vi "ACC_MANAGEMENT.vi"() -> ()   [LabVIEW 2018]
uses:
  <vilib>/addons/database/Connection.llb/DB Tools Open Connec (Path).vi
  <vilib>/addons/database/Connection.llb/Conn Execute.vi
  <vilib>/addons/database/Recordset.llb/Rec Fetch Recordset Data (R).vi
  <vilib>/addons/database/Recordset.llb/Rec Destroy - Connection.vi
  <vilib>/addons/database/_DB Variant To Data/Database Variant To Data.xnode
  <vilib>/addons/database/NI_Database_API.lvlib
panel:
  in  "MAIN_TAB":T1(tab)
  in  "ACC_PASSPORT_VALID":string caption="NEW PASSWORD"
  in  "ACC_SAVE":bool
  in  "ACC_IMG_UP":bool
  in  "ACC_STAMP":string caption="SUPPORTING"
  in  "ACC_TITLE":string caption="NEW PASSWORD"
  in  "ACC_UNIT":string caption="NEW PASSWORD"
  in  "ACC_EMAIL":string caption="NEW PASSWORD"
  in  "ACC_NAME":string caption="NEW PASSWORD"
  in  "ACC_UID":string caption="CONFIRM NEW PASSWORD"
  out "ACC_ACCESS":string[][](table)
  in  "ACC_BUTTON1":bool
  in  "ACC_PSW2":string caption="CONFIRM PASSWORD"
  in  "ACC_PSW1":string caption="NEW PASSWORD"
  in  "ACC_OPTION":enum32{"Item 0", "Item 1", "Item 2"}(radio)
  out "ACC_IMG":picture
  in  "ACC_IMG_DN":bool
  in  "ACC_BUTTON2":bool
  in  "ACC_STAMP_STATUS":bool
  out "ACC_STATUS":bool caption="TRANSACTION SUCCESS"
  in  "ACC_TAG":u16(ring) items=["BARCODE", "RFID", "NFC"]
  out "ACC_TAG_ID":string caption="NEW PASSWORD"
  in  "ACC_PASSPORT_UP":bool
  in  "ACC_PASSPORT_DN":bool
  in  "ACC_PASSPORT":string caption="NEW PASSWORD"
  in  "ACC_PASSPORT_TIMESTAMP":timestamp format="%<%b %d, %Y>T"
  in  "ACC_PASSPORT_STATUS":bool
  in  "MNG_MODULE_ACC":u16(ring) items=["R", "R/W", "R/W/D"]
  in  "MNG_MODULE":i32(listbox)
  in  "MNG_KEYWORD":string
  in  "MNG_SELECT":u16(ring) items=["by UID", "by NAME", "by EMAIL"]
  out "MNG_STATUS":bool
  in  "MNG_SRC/DLT":bool
  in  "MNG_MODULE_UPD":bool
  out "MAIN_NOTE":string caption="ADDITIONAL NOTE :"
  in  "MAIN_CLOSE":bool
  in  "MAIN_LOGIN":string
  # "ACCOUNT MANAGEMENT"
  # "UID :"
  # "PSW :"
  # "BASIC INFORMATION"
  # "NAME   :"
  # "EMAIL  :"
  # "UNIT   :"
  # "TITLE  :"
  # "STAMP  :"
  # "SMART TAG"
  # ":"
  # "TRAVEL DOCUMENT"
  # "PASSPORT    :"
  # "VALID UNTIL :"
  # "ACCESSIBILITY :"
  # "KEYWORD :"
  # "ACCESSIBILITY :"
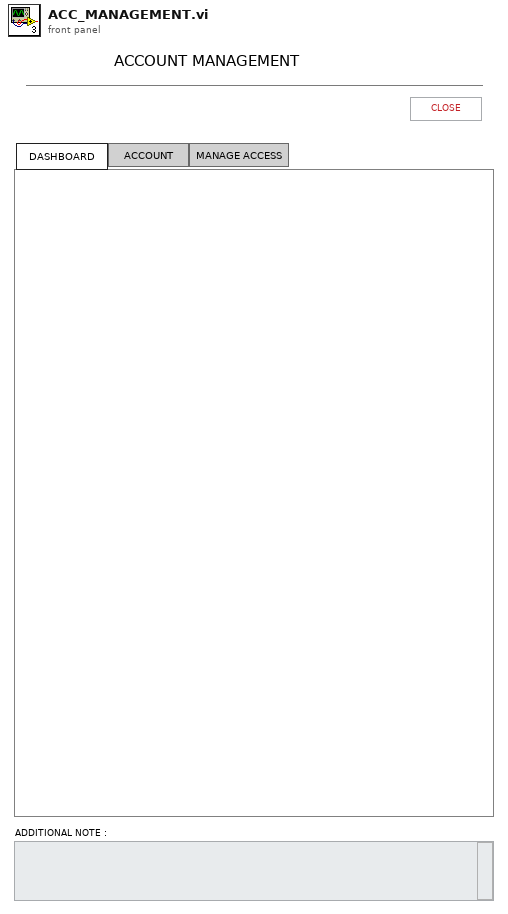
[diagram p1: front panel]
types:
  T1 = enum32{"DASHBOARD    ", "ACCOUNT      ", "MANAGE ACCESS"}
  T2 = enum16{"open", "replace", "create", "open or create", "replace or create", "replace or create with confirmation"}
  T3 = enum8{"Enabled", "Disabled", "Disabled and Grayed Out"}
  T4 = typedef "NI_Database_API.lvlib/Conn ObjectReference.ctl" = refnum<k1>
  T5 = typedef "NI_Database_API.lvlib/Rec ObjectReference.ctl" = refnum<k1>
  T6 = cluster{string[], string[], string[], string[], string[], path, path}
  T7 = typedef "LVBoundsTypeDef.ctl" = cluster{"Width":u32, "Height":u32}
  T8 = typedef "imagedata.ctl" = cluster{"image type":i32, "image depth":i32, "image":u8[], "mask":u8[], "colors":u32[], "Rectangle":cluster{"left":i16, "top":i16, "right":i16, "bottom":i16}}
  T9 = cluster{string[], string[], string[], string[], string[], "new picture":picture, dbl, bool}
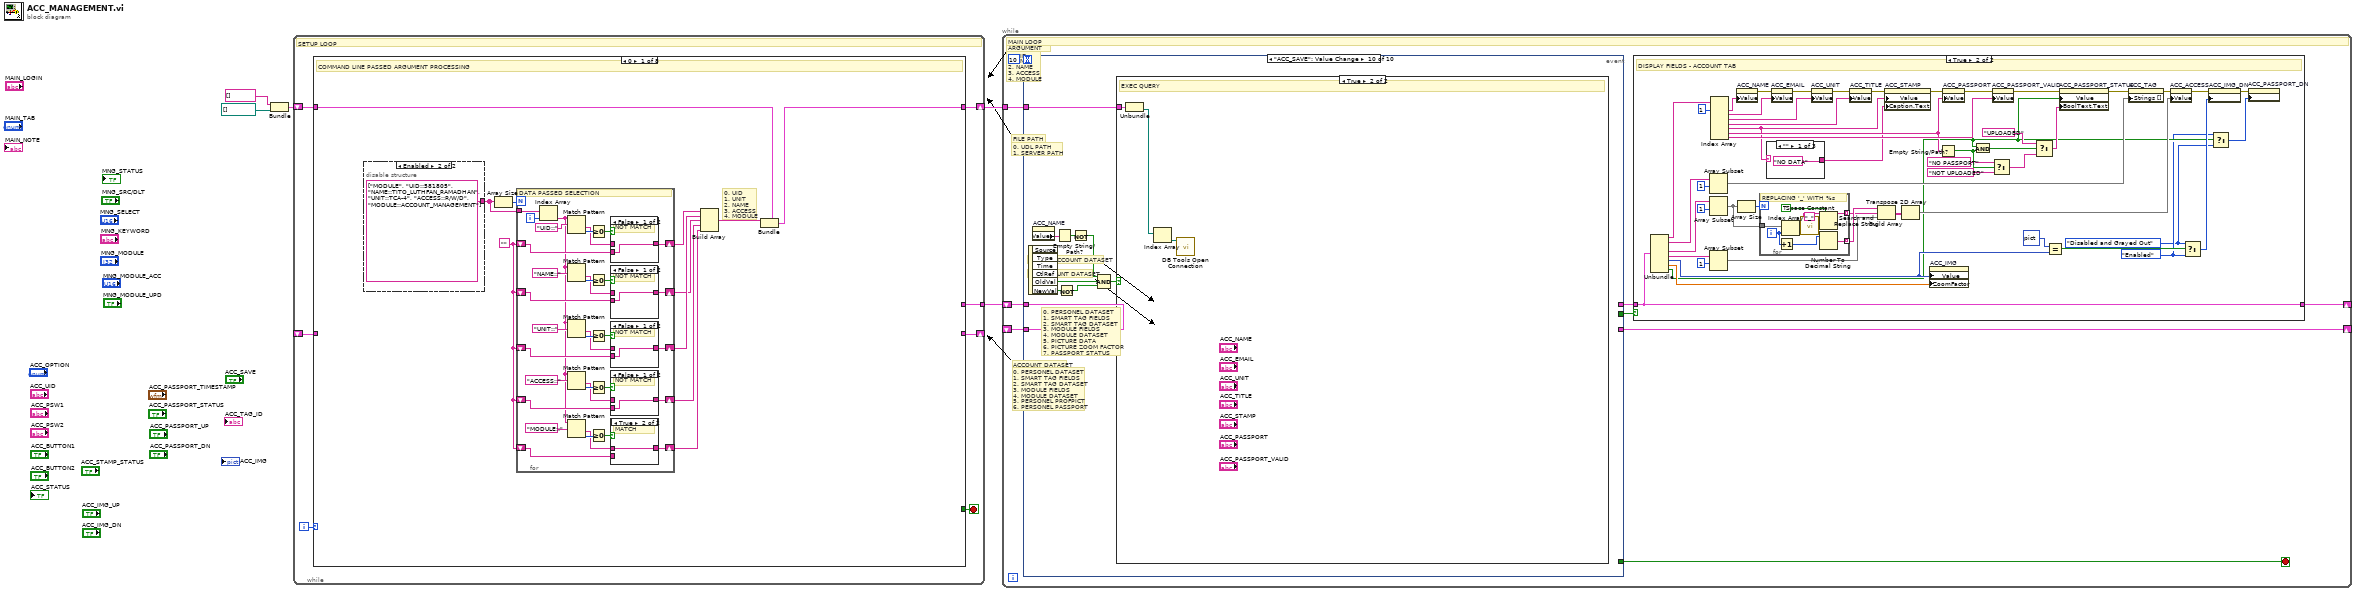
[diagram p0: block diagram]
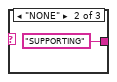
[diagram p3: hidden frame]
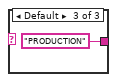
[diagram p4: hidden frame]
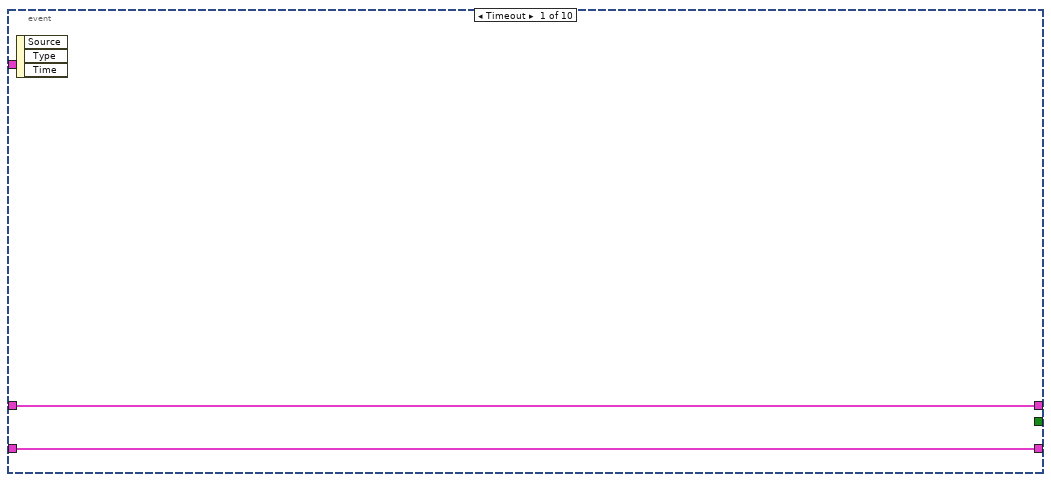
[diagram p5: hidden frame]
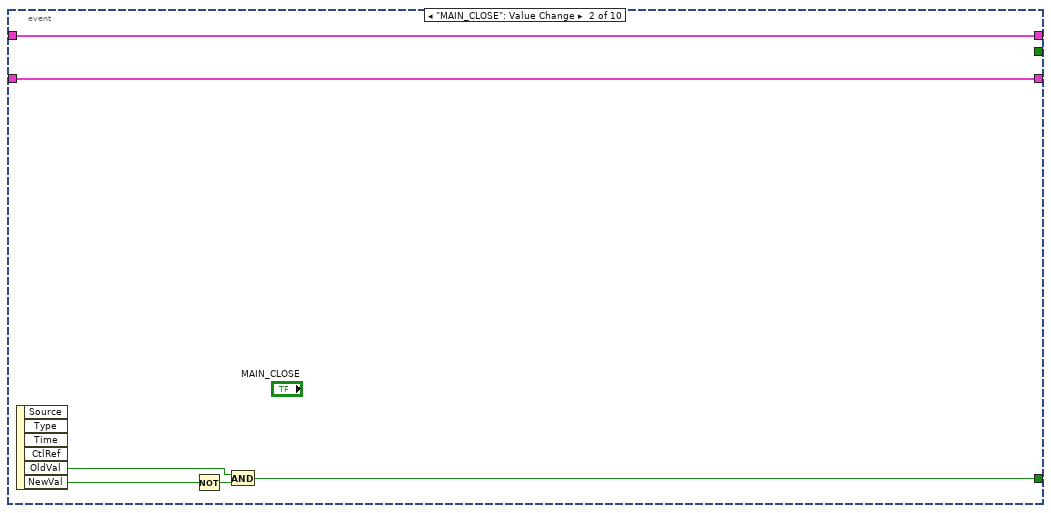
[diagram p6: hidden frame]
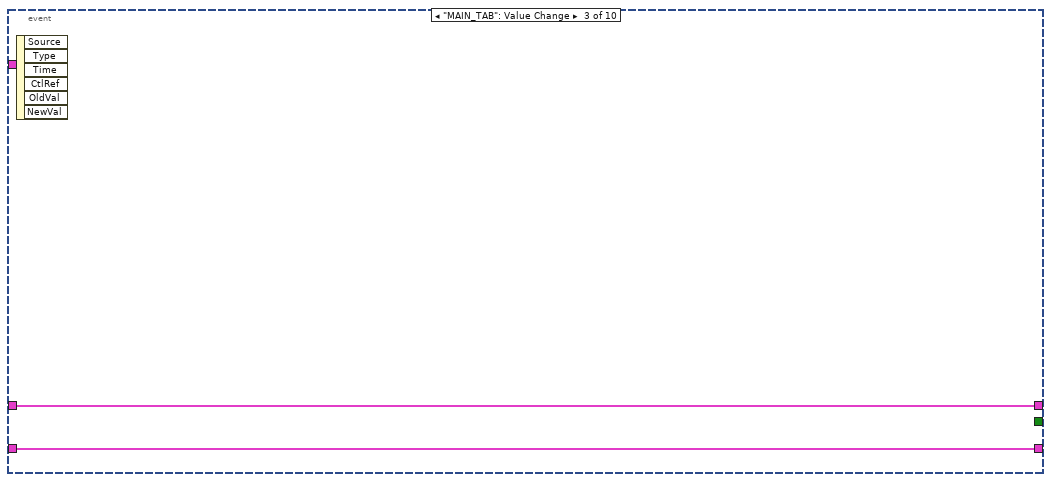
[diagram p7: hidden frame]
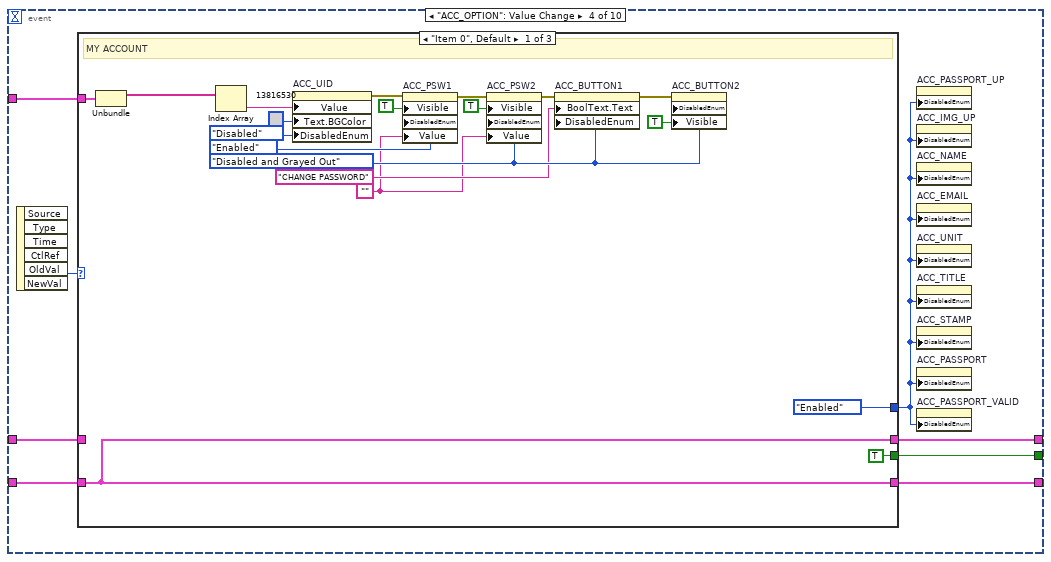
[diagram p8: hidden frame]
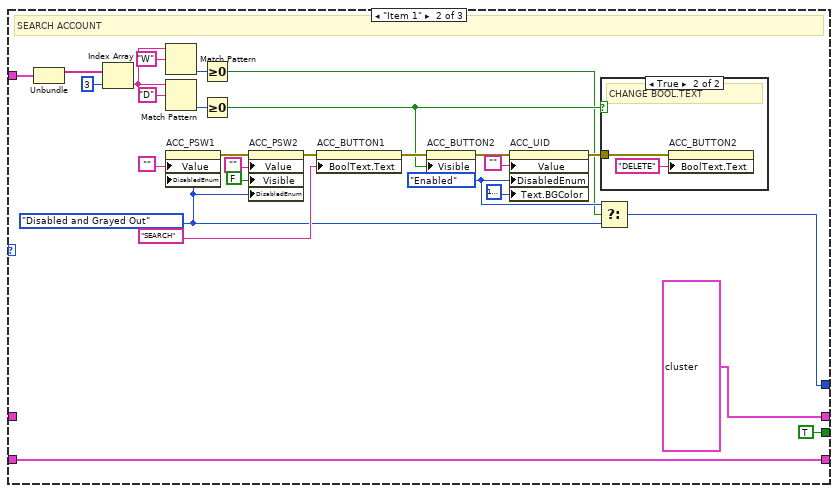
[diagram p9: hidden frame]
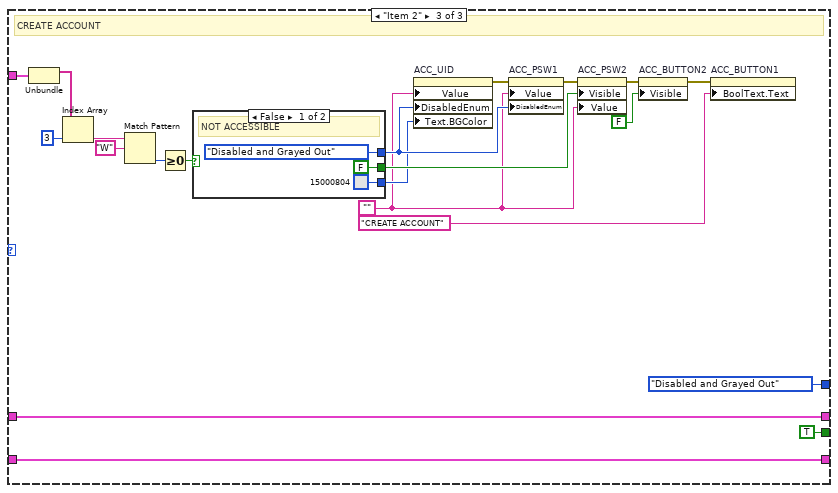
[diagram p11: hidden frame]
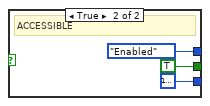
[diagram p12: hidden frame]
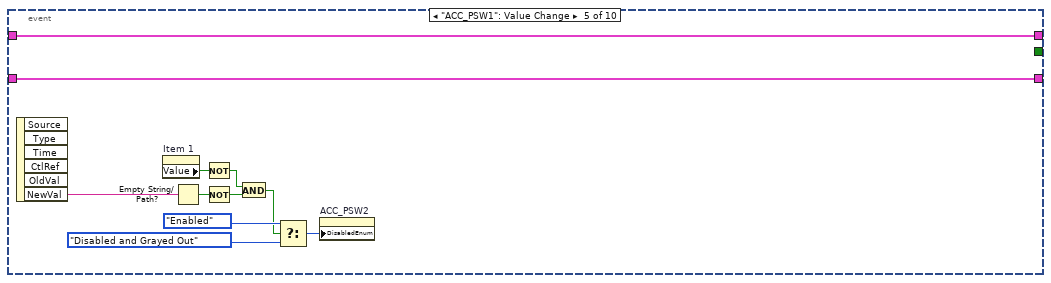
[diagram p13: hidden frame]
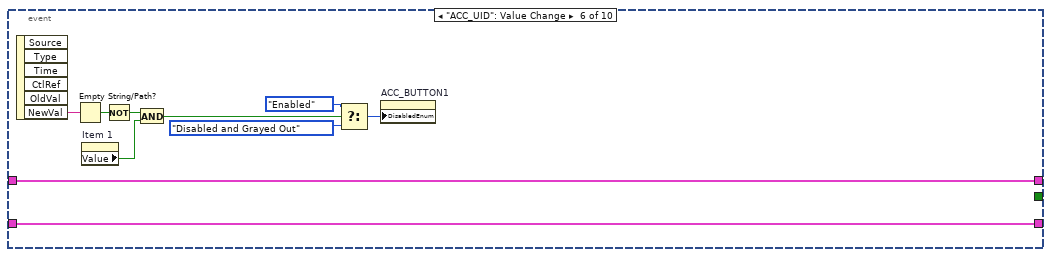
[diagram p14: hidden frame]
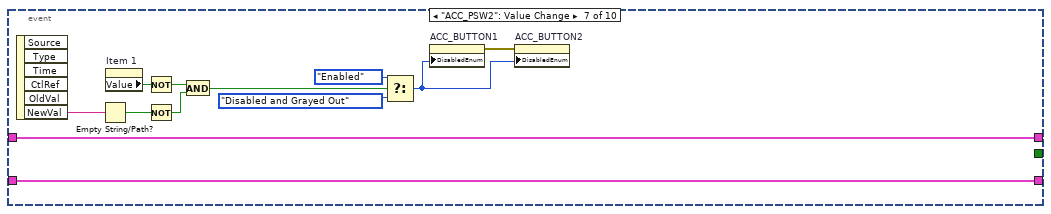
[diagram p15: hidden frame]
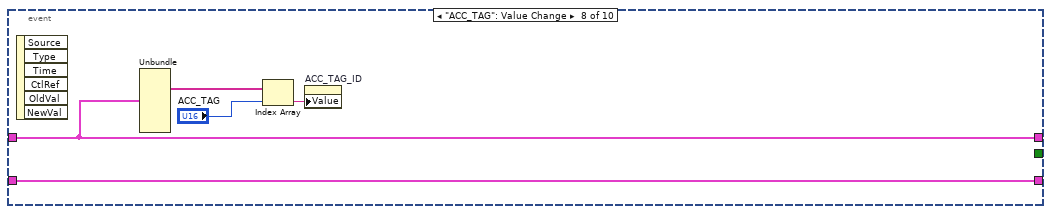
[diagram p16: hidden frame]
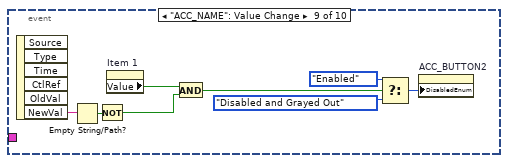
[diagram p17: hidden frame]
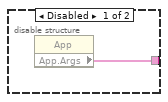
[diagram p19: hidden frame]
diagram:
  # "MY ACCOUNT DATASET"
  # "0. PERSONEL DATASET\n1. SMART TAG FIELDS\n2. SMART TAG DATASET\n3. MODULE FIELDS\n4. MODULE DATASET\n5. PICTURE DATA\n6. PICTURE ZOOM FACTOR\n7. PASSPORT STATUS"
  # "OTHER ACCOUNT DATASET"
  # "0. PERSONEL DATASET\n1. SMART TAG FIELDS\n2. SMART TAG DATASET\n3. MODULE FIELDS\n4. MODULE DATASET\n5. PERSONEL PROFPICT\n6. PERSONEL PASSPORT"
  # "0. UDL PATH\n1. SERVER PATH"
  # "0. UID\n1. UNIT\n2. NAME\n3. ACCESS\n4. MODULE"
  # "ACCOUNT DATASET"
  # "FILE PATH"
  # "COMMAND LINE\nARGUMENT"
  n1 = Bundle(string[] [], path[] []) -> (w3:cluster{string[], path[]})  [unwired: 1 in]
  n2 = while {
    shift-right: [w11] -> _
    shift-left: _ -> [w10]
    tunnel: [w8] -> w1
    shift-right: [w7] -> w2
    shift-left: w3 -> [w6]
    i -> [w12]
    stop <- w9 stop-if-true
    # "SETUP LOOP"
    n3 = case shown="0" w12 {
      tunnel: [_ _ _ w163 _ _ _ TRUE] -> w9
      tunnel: [_ _ _ w157 w405 w500 w523 w532] -> w11
      tunnel: w10 -> [_ _ _ w156 w405 w500 w523 w532]
      tunnel: [_ _ _ _ _ _ _ w531] -> w8
      tunnel: w6 -> [w15 w73 w98 w155 w404 w408 w522 w530]
      tunnel: [w13 w73 w96 w155 w404 w408 w522 w530] -> w7
      frame 0 {
        w21 = ""
        # "0. UID\n1. UNIT\n2. NAME\n3. ACCESS\n4. MODULE"
        # "COMMAND LINE PASSED ARGUMENT PROCESSING"
        n4 = disable-structure shown="Enabled" {
          disable-tunnel: [w24 string[] ["MODULE", "UID::581805", "NAME::TITO_LUTHFAN_RAMADHAN", "UNIT::TCA-4", "ACCESS::R/W/D", "MODULE::ACCOUNT_MANAGEMENT"] ("App.Args")] -> w22
          frame Disabled {
            n5 = property class="App"() -> ("App.Args"=w24:string[])  [unwired: 2 in, 2 out]
          }
          frame Enabled {
          }
        }
        n6 = Array Size(array=w22) -> (size(s)=w23:i32)
        n7 = for {
          N: w23 -> [_]
          tunnel: w22 -> [w58]
          shift-right: [w52] -> w19
          shift-left: w21 -> [w47]
          shift-right: [w46] -> w17
          shift-left: w21 -> [w45]
          shift-right: [w41] -> w18
          shift-left: w21 -> [w39]
          shift-right: [w34] -> w16
          shift-left: w21 -> [w33]
          shift-right: [w28] -> w20
          shift-left: w21 -> [w27]
          i -> [w57]
          # "DATA PASSED SELECTION"
          n8 = Index Array(array=w58, index=w57) -> (element=w26:string)
          n9 = Match Pattern(string=w26, regular expression="UID::") -> (after substring=w53:string, offset past match=w55:i32)  [unwired: 1 in, 2 out]
          n10 = Match Pattern(string=w26, regular expression="NAME::") -> (after substring=w48:string, offset past match=w51:i32)  [unwired: 1 in, 2 out]
          n11 = Match Pattern(string=w26, regular expression="UNIT::") -> (after substring=w40:string, offset past match=w44:i32)  [unwired: 1 in, 2 out]
          n12 = Match Pattern(string=w26, regular expression="ACCESS::") -> (after substring=w35:string, offset past match=w37:i32)  [unwired: 1 in, 2 out]
          n13 = Match Pattern(string=w26, regular expression="MODULE::") -> (after substring=w29:string, offset past match=w31:i32)  [unwired: 1 in, 2 out]
          n14 = Greater Or Equal To 0?(x=w55) -> (x >= 0?=w54:bool)
          n15 = Greater Or Equal To 0?(x=w51) -> (x >= 0?=w50:bool)
          n16 = Greater Or Equal To 0?(x=w44) -> (x >= 0?=w43:bool)
          n17 = Greater Or Equal To 0?(x=w37) -> (x >= 0?=w38:bool)
          n18 = Greater Or Equal To 0?(x=w31) -> (x >= 0?=w32:bool)
          n19 = case shown="False" w54 {
            tunnel: [w71 w72] -> w52
            tunnel: w53 -> [_ w72]
            tunnel: w47 -> [w71 _]
            frame False {
              # "NOT MATCH"
            }
            frame True {
              # "MATCH"
            }
          }
          n20 = case shown="False" w50 {
            tunnel: [w65 w66] -> w46
            tunnel: w48 -> [_ w70]
            tunnel: w45 -> [w65 _]
            frame False {
              # "NOT MATCH"
            }
            frame True {
              # "MATCH"
              n21 = call <vilib>:"Space Constant.vi"() -> ("String"=w68:string)
              n22 = Search and Replace String(replace all?=TRUE ("replace all? (F)"), input string=w70, search string="_", replace string=w68) -> (result string=w66:string)  [unwired: 4 in, 3 out]
            }
          }
          n23 = case shown="False" w43 {
            tunnel: [w63 w64] -> w41
            tunnel: w40 -> [_ w64]
            tunnel: w39 -> [w63 _]
            frame False {
              # "NOT MATCH"
            }
            frame True {
              # "MATCH"
            }
          }
          n24 = case shown="False" w38 {
            tunnel: [w61 w62] -> w34
            tunnel: w35 -> [_ w62]
            tunnel: w33 -> [w61 _]
            frame False {
              # "NOT MATCH"
            }
            frame True {
              # "MATCH"
            }
          }
          n25 = case shown="True" w32 {
            tunnel: [w59 w60] -> w28
            tunnel: w29 -> [_ w60]
            tunnel: w27 -> [w59 _]
            frame False {
              # "NOT MATCH"
            }
            frame True {
              # "MATCH"
            }
          }
        }
        n26 = Build Array(w19, w18, w17, w16, w20) -> (w14:string[])
        n27 = Bundle(cluster=w15, w14) -> (w13:cluster{string[], path[]})  [unwired: 1 in]
      }
      frame 1 {
        w82 = " | " ("string")
        # "0. UID\n1. UNIT\n2. NAME\n3. ACCESS\n4. MODULE"
        # "INITIALIZE UI; SET FRONT PANEL SIZE AND POSITION; SET INITIAL VALUE FOR TITLE SECTION"
        n28 = Unbundle(w73) -> (w74:string[])  [unwired: 1 out]
        n29 = control-ref of="This VI"() -> (w92:refnum<vi>)
        n30 = Index Array(array=w74) -> (element #1=w78:string, element #2=w77:string, element #3=w76:string, element #4=w75:string)  [unwired: 5 in, 1 out]
        n31 = invoke class="VI" method="Default Vals.Reinit All"(reference=w92) -> (reference out=w91:refnum<vi>, error out=w90:errorcluster)  [unwired: 2 in, 1 out]
        n32 = case shown="\"R/W/D\"" w75 {
          tunnel: ["STANDARD USER" "SUPER USER" "ADMINISTRATOR"] -> w83
          frame "R", Default {
            # "READ ONLY"
          }
          frame "R/W" {
            # "READ; WRITE"
          }
          frame "R/W/D" {
            # "READ; WRITE; DELETE"
          }
        }
        n33 = Concatenate Strings(w78, w82, w77, w82, w76, "\r\n", "ACCESS : " ("string"), w83) -> (w84:string)
        n34 = invoke class="VI" method="FP.Run-Time Position.Custom"(reference=w91, error in=w90, "Size"=cluster{"Top":i16, "Left":i16} {"Top"=0, "Left"=383} ("Position"), "Position"=cluster{"Height":i16, "Width":i16} {"Height"=888, "Width"=505} ("Size")) -> (reference out=w86:refnum<vi>, error out=w87:errorcluster)  [unwired: 1 in, 3 out]
        n35 = Close Reference(reference=w86, error in (no error)=w87) -> (error out=w85:errorcluster)
        n36 = call <vilib>:"Clear Errors.vi"("error in (no error)"=w85) -> ("error out"=w79:errorcluster)  [unwired: 5 in, 1 out]
        n37 = property on="MAIN_LOGIN" class="Str"(error in=w79, "Value"=w84) -> ()  [unwired: 1 in, 2 out]
      }
      frame 2 {
        # "0. UDL PATH\n1. SERVER PATH"
        # "GET FILE PATHS NEEDED"
        n38 = disable-structure shown="Enabled" {
          disable-tunnel: [_ w100] -> w97
          frame Disabled {
            w99 = path "D:/Coding/AVIONICS PORTAL/CONNECT/CONSTR_#1_PERSONEL_ADMIN.udl" ("connection information")
          }
          frame Enabled {
            n39 = call <vilib>:"Application Directory.vi"() -> ("Application Directory"=w124:path)
            n40 = Path To String(path=w124) -> (string=w123:string)
            n41 = Match Pattern(string=w123, regular expression="MODULES\\") -> (before substring=w121:string)  [unwired: 1 in, 3 out]
            n42 = Concatenate Strings(w121, "CONNECT\\") -> (w114:string)
            n43 = String To Path(string=w114) -> (path=w119:path)
            n44 = List Folder(path=w119) -> (filenames=w116:string[])  [unwired: 3 in, 3 out]
            n45 = Array Size(array=w116) -> (size(s)=w117:i32)
            n46 = while {
              tunnel: w116 -> [w152]
              tunnel: w117 -> [w147]
              tunnel: [w140] -> w118
              i -> [w145]
              stop <- w143 stop-if-true
              # "POINTING CONSTR #1"
              n47 = Index Array(array=w152, index=w145) -> (element=w151:string)
              n48 = Decrement(x=w147) -> (x-1=w146:i32)
              n49 = Match Pattern(string=w151, regular expression="CONSTR#1") -> (before substring=w139:string, match substring=w142:string, after substring=w141:string, offset past match=w149:i32)  [unwired: 1 in]
              n50 = Equal?(x=w146, y=w145) -> (x = y?=w144:bool)
              n51 = Greater Or Equal To 0?(x=w149) -> (x >= 0?=w148:bool)
              n52 = Or(x=w144, y=w148) -> (x .or. y?=w143:bool)
              n53 = Concatenate Strings(w139, w142, w141) -> (w140:string)
            }
            n54 = while {
              tunnel: w116 -> [w138]
              tunnel: w117 -> [w133]
              tunnel: [w126] -> w113
              i -> [w131]
              stop <- w129 stop-if-true
              # "POINTING CONSTR #1"
              n55 = Index Array(array=w138, index=w131) -> (element=w137:string)
              n56 = Decrement(x=w133) -> (x-1=w132:i32)
              n57 = Match Pattern(string=w137, regular expression="PATH#1") -> (before substring=w125:string, match substring=w128:string, after substring=w127:string, offset past match=w135:i32)  [unwired: 1 in]
              n58 = Equal?(x=w132, y=w131) -> (x = y?=w130:bool)
              n59 = Greater Or Equal To 0?(x=w135) -> (x >= 0?=w134:bool)
              n60 = Or(x=w130, y=w134) -> (x .or. y?=w129:bool)
              n61 = Concatenate Strings(w125, w128, w127) -> (w126:string)
            }
            n62 = Concatenate Strings(w114, w118) -> (w115:string)
            n63 = Concatenate Strings(w114, w113) -> (w112:string)
            n64 = String To Path(string=w115) -> (path=w102:path)
            n65 = String To Path(string=w112) -> (path=w111:path)
            n66 = Open/Create/Replace File(file path (use dialog)=w111, operation (0:open)=T2."open", access (0:read/write)=enum16{"read/write", "read-only", "write-only"}."read-only") -> (refnum out=w108:refnum<file>, error out=w109:errorcluster)  [unwired: 3 in, 1 out]
            n67 = Read from Text File(file (use dialog)=w108, error in=w109) -> (refnum out=w105:refnum<file>, text=w107:string, error out=w106:errorcluster)  [unwired: 2 in, 1 out]
            n68 = String To Path(string=w107) -> (path=w101:path)
            n69 = Close File(refnum=w105, error in=w106) -> (error out=w104:errorcluster)  [unwired: 1 out]
            n70 = Build Array(w102, w101) -> (w100:path[])
            n71 = call <vilib>:"Clear Errors.vi"("error in (no error)"=w104) -> ()  [unwired: 5 in, 2 out]
          }
        }
        n72 = Bundle(cluster=w98, w97) -> (w96:cluster{string[], path[]})  [unwired: 1 in]
      }
      frame 3 {
        # "RETRIEVE ACCOUNT DATASET FROM DATABASE; RETRIEVE FILEPATH FOR IMAGE; RETRIEVE FILEPATH FOR PASSPORT"
        n73 = Unbundle(w155) -> (w153:string[], w154:path[])
        n74 = Index Array(array=w154, index #1=0 ("index"), index #2=1 ("index")) -> (element #1=w160:path, element #2=w158:path)
        n75 = call-poly <vilib>:"DB Tools Open Connection.vi"("connection information"=w160) -> ("error out"=w164:errorcluster, "connection reference"=w162:T4)  [unwired: 7 in]
        n76 = case shown="No Error" w164 {
          selector: w164 -> [w228 w397]
          tunnel: [_ w400] -> w163
          tunnel: w162 -> [w229 _]
          tunnel: w160 -> [_ w403]
          tunnel: w153 -> [w249 _]
          tunnel: w158 -> [w189 _]
          tunnel: w153 -> [w186 _]
          tunnel: [w173 w396] -> w157
          tunnel: w156 -> [_ w396]
          frame No Error {
            w183 = "\\" ("string")
            w199 = string[][] []
            w204 = "';" ("string")
            # "PROFPICT FILEPATH"
            # "PASSPORT FILEPATH"
            # "MODULE DATASET"
            # "MODULE FIELDS"
            # "SMART TAG DATASET"
            # "SMART TAG FIELDS"
            # "PERSONEL DATASET"
            # "0. PERSONEL DATASET\n1. SMART TAG FIELDS\n2. SMART TAG DATASET\n3. MODULE FIELDS\n4. MODULE DATASET\n5. PERSONEL PROFPICT\n6. PERSONEL PASSPORT"
            n77 = Path To String(path=w189) -> (string=w188:string)
            n78 = Index Array(array=w186, index=4) -> (element=w184:string)
            n79 = Index Array(array=w249, index=0) -> (element=w181:string)
            n80 = call <vilib>:"DB Tools List Columns.vi"("error in (no error)"=w228, "table"="login", "connection reference"=w229) -> ("error out"=w226:errorcluster, "columns"=w219:string[], "connection reference out"=w227:T4)  [unwired: 1 in, 1 out]
            n81 = Concatenate Strings(w181, "_PROFPICT.jpg" ("string")) -> (w179:string)
            n82 = Concatenate Strings(w181, "_PASSPORT.pdf" ("string")) -> (w177:string)
            n83 = Concatenate Strings(w188, "\\MODULE\\" ("string"), w184, w183, w181, w183) -> (w178:string)
            n84 = Concatenate Strings("SELECT * FROM smart_tag WHERE UID = '", w181, w204) -> (w203:string)
            n85 = Concatenate Strings("SELECT * FROM login WHERE UID = '", w181, w204) -> (w230:string)
            n86 = Concatenate Strings("SELECT * FROM personel WHERE UID = '", w181, w204) -> (w246:string)
            n87 = call <vilib>:"DB Tools List Columns.vi"("error in (no error)"=w226, "table"="smart_tag", "connection reference"=w227) -> ("error out"=w224:errorcluster, "columns"=w221:string[], "connection reference out"=w225:T4)  [unwired: 1 in, 1 out]
            n88 = call-poly <vilib>:"DB Tools Execute Query.vi"("error in (no error)"=w224, "SQL query"=w246, "connection reference"=w225) -> ("error out"=w245:errorcluster, "recordset reference"=w244:T5)  [unwired: 5 in]
            n89 = Concatenate Strings(w178, w179) -> (w176:string)
            n90 = Concatenate Strings(w178, w177) -> (w175:string)
            n91 = Array Subset(array=w221, index=1) -> (w216:string[])  [unwired: 1 in]
            n92 = Array Subset(array=w219, index=2) -> (w214:string[])  [unwired: 1 in]
            n93 = call-poly <vilib>:"DB Tools Fetch Recordset Data.vi"("error in (no error)"=w245, "recordset reference"=w244) -> ("error out"=w242:errorcluster, "recordset data"=w243:variant[][], "recordset reference out"=w241:T5)  [unwired: 3 in]
            n94 = String To Path(string=w176) -> (path=w172:path)
            n95 = String To Path(string=w175) -> (path=w174:path)
            n96 = xnode "Database Variant To Data"("database variant"=w243, "type"=w199) -> ("data"=w240:string[][])  [unwired: 1 in, 1 out]
            n97 = Array Size(array=w216) -> (size(s)=w217:i32)
            n98 = Array Size(array=w214) -> (size(s)=w215:i32)
            n99 = call-poly <vilib>:"DB Tools Free Object.vi"("error in (no error)"=w242, "recordset reference"=w241) -> ("error out"=w165:errorcluster, "connection reference"=w237:T4)  [unwired: 8 in]
            n100 = call <vilib>:"Clear Errors.vi"("error in (no error)"=w165) -> ("error out"=w166:errorcluster)  [unwired: 5 in, 1 out]
            n101 = call-poly <vilib>:"DB Tools Execute Query.vi"("error in (no error)"=w166, "SQL query"=w230, "connection reference"=w237) -> ("error out"=w236:errorcluster, "recordset reference"=w235:T5)  [unwired: 5 in]
            n102 = Index Array(array=w240, index (row)=0) -> (element=w171:string[])  [unwired: 1 in]
            n103 = for {
              N: w215 -> [_]
              tunnel: w214 -> [w299]
              tunnel: [w294] -> w191 mode=indexing
              i -> [w300]
              # "REPLACE '_' WITH %s"
              n104 = Index Array(array=w299, index=w300) -> (element=w298:string)
              n105 = call <vilib>:"Space Constant.vi"() -> ("String"=w295:string)
              n106 = Search and Replace String(replace all?=TRUE ("replace all? (F)"), input string=w298, search string="_", replace string=w295) -> (result string=w294:string)  [unwired: 4 in, 3 out]
            }
            n107 = for {
              N: w217 -> [_]
              tunnel: w216 -> [w306]
              tunnel: [w301] -> w197 mode=indexing
              i -> [w307]
              # "REPLACE '_' WITH %s"
              n108 = Index Array(array=w306, index=w307) -> (element=w305:string)
              n109 = call <vilib>:"Space Constant.vi"() -> ("String"=w302:string)
              n110 = Search and Replace String(replace all?=TRUE ("replace all? (F)"), input string=w305, search string="_", replace string=w302) -> (result string=w301:string)  [unwired: 4 in, 3 out]
            }
            n111 = Array Subset(array=w171, index=1) -> (w169:string[])  [unwired: 1 in]
            n112 = call-poly <vilib>:"DB Tools Fetch Recordset Data.vi"("error in (no error)"=w236, "recordset reference"=w235) -> ("error out"=w233:errorcluster, "recordset data"=w232:variant[][], "recordset reference out"=w234:T5)  [unwired: 3 in]
            n113 = call-poly <vilib>:"DB Tools Free Object.vi"("error in (no error)"=w233, "recordset reference"=w234) -> ("error out"=w168:errorcluster, "connection reference"=w208:T4)  [unwired: 8 in]
            n114 = xnode "Database Variant To Data"("database variant"=w232, "type"=w199) -> ("data"=w207:string[][])  [unwired: 1 in, 1 out]
            n115 = call <vilib>:"Clear Errors.vi"("error in (no error)"=w168) -> ("error out"=w167:errorcluster)  [unwired: 5 in, 1 out]
            n116 = call-poly <vilib>:"DB Tools Execute Query.vi"("error in (no error)"=w167, "SQL query"=w203, "connection reference"=w208) -> ("error out"=w213:errorcluster, "recordset reference"=w212:T5)  [unwired: 5 in]
            n117 = Index Array(array=w207, index (row)=0) -> (element=w193:string[])  [unwired: 1 in]
            n118 = Array Subset(array=w193, index=2) -> (w190:string[])  [unwired: 1 in]
            n119 = call-poly <vilib>:"DB Tools Fetch Recordset Data.vi"("error in (no error)"=w213, "recordset reference"=w212) -> ("error out"=w210:errorcluster, "recordset data"=w209:variant[][], "recordset reference out"=w211:T5)  [unwired: 3 in]
            n120 = call-poly <vilib>:"DB Tools Free Object.vi"("error in (no error)"=w210, "recordset reference"=w211) -> ("error out"=w201:errorcluster, "connection reference"=w202:T4)  [unwired: 8 in]
            n121 = xnode "Database Variant To Data"("database variant"=w209, "type"=w199) -> ("data"=w200:string[][])  [unwired: 1 in, 1 out]
            n122 = call <vilib>:"DB Tools Close Connection.vi"("error in (no error)"=w201, "connection reference"=w202) -> ("error out"=w238:errorcluster)  [unwired: 5 in]
            n123 = Index Array(array=w200, index (row)=0) -> (element=w196:string[])  [unwired: 1 in]
            n124 = Array Subset(array=w196, index=1) -> (w194:string[])  [unwired: 1 in]
            n125 = call <vilib>:"Clear Errors.vi"("error in (no error)"=w238) -> ()  [unwired: 5 in, 2 out]
            n126 = Bundle(w169, w197, w194, w191, w190, w172, w174) -> (w173:T6)  [unwired: 1 in]
          }
          frame Error {
            n127 = Path To String(path=w403) -> (string=w398:string)
            n128 = call <vilib>:"Clear Errors.vi"("error in (no error)"=w397) -> ()  [unwired: 5 in, 2 out]
            n129 = Concatenate Strings("FATAL ERROR!\nCONNECTION REFERENCE IS NOT ACCESSIBLE.\n\n" ("string"), w398) -> (w402:string)
            n130 = One Button Dialog(message=w402, button name ("OK")="QUIT") -> (true=w400:bool)
          }
        }
      }
      frame 4 {
        # "DASHBOARD PAGE SETUP"
      }
      frame 5 {
        w424 = TRUE
        w425 = T3."Disabled and Grayed Out" ("Disabled")
        # "0. PERSONEL DATASET\n1. SMART TAG FIELDS\n2. SMART TAG DATASET\n3. MODULE FIELDS\n4. MODULE DATASET\n5. PERSONEL PROFPICT\n6. PERSONEL PASSPORT"
        # "PERSONEL PROFTPICT"
        # "ACCOUNT PAGE SETUP"
        n131 = Unbundle(w408) -> (w407:string[])  [unwired: 1 out]
        n132 = Unbundle(w500) -> (w498:string[], w458:string[], w452:string[], w441:string[], w445:string[], w499:path, w488:path)
        n133 = Index Array(array=w498) -> (element #1=w469:string, element #2=w497:string, element #3=w496:string, element #4=w495:string, element #5=w494:string, element #6=w433:string, element #7=w484:string, element #8=w412:string, element #9=w474:string, element #10=w472:string)  [unwired: 10 in]
        n134 = Index Array(array=w407, index=0) -> (element=w436:string)
        n135 = Empty String/Path?(string/path=w469) -> (empty?=w466:bool)
        n136 = Not(x=w466) -> (.not. x?=w467:bool)
        n137 = Select(t=u32 16742513, s=w466, f=u32 16777222) -> (s? t:f=w463:u32)
        n138 = Select(t="TRANSACTION FAILED!", s=w466, f="TRANSACTION SUCCESS ") -> (s? t:f=w462:string)
        n139 = property on="ACC_IMG" class="Pict"() -> (error out=w418:errorcluster, "Draw Area Size"=w511:T7)  [unwired: 2 in, 1 out]
        n140 = call <vilib>:"Read JPEG File.vi"("path to JPEG file"=w499) -> ("error out"=w417:errorcluster, "image data"=w502:T8)  [unwired: 8 in, 1 out]
        n141 = property on="ACC_STATUS" class="Bool (strict)"("Caption.TextColor"=w463, "Caption.Text"=w462, "Value"=w467) -> (error out=w477:errorcluster)  [unwired: 2 in, 1 out]
        n142 = Index Array(array=w452, index #1=0 ("index")) -> (element #1=w456:string, element #2=w409:string)  [unwired: 1 in]
        n143 = Index Array(array=w445, index=0) -> (element=w443:string)
        n144 = Array Subset(array=w458, index=1) -> (w459:string[])  [unwired: 1 in]
        n145 = Array Subset(array=w441, index=1) -> (w440:string[])  [unwired: 1 in]
        n146 = Array Subset(array=w445, index=1) -> (w446:string[])  [unwired: 1 in]
        n147 = Array Size(array=w440) -> (size(s)=w453:i32)
        n148 = Unbundle By Name(w511) -> ("Width"=w510:u32, "Height"=w508:u32)
        n149 = Unbundle By Name(w502) -> ("Rectangle.right"=w509:i16, "Rectangle.bottom"=w507:i16)
        n150 = call <vilib>:"Draw Flattened Pixmap.vi"("image data"=w502) -> ("new picture"=w501:picture)  [unwired: 8 in]
        n151 = call <vilib>:"Clear Errors.vi"("error in (no error)"=w417) -> ("error out"=w413:errorcluster)  [unwired: 5 in, 1 out]
        n152 = for {
          N: w453 -> [_]
          tunnel: w440 -> [w521]
          tunnel: [w516] -> w450 mode=indexing
          tunnel: [w513] -> w451 mode=indexing
          i -> [w515]
          # "REPLACING '_' WITH %s"
          n153 = Increment(x=w515) -> (x+1=w514:i32)
          n154 = Index Array(array=w521, index=w515) -> (element=w520:string)
          n155 = call <vilib>:"Space Constant.vi"() -> ("String"=w518:string)
          n156 = Search and Replace String(replace all?=TRUE, input string=w520, search string="_", replace string=w518) -> (result string=w516:string)  [unwired: 4 in, 3 out]
          n157 = Number To Decimal String(number=w514) -> (decimal integer string=w513:string)  [unwired: 1 in]
        }
        n158 = property on="ACC_NAME" class="Str"(error in=w477, "Value"=w497) -> (error out=w493:errorcluster)  [unwired: 1 in, 1 out]
        n159 = Select(t=2, s=w417, f=0) -> (s? t:f=w414:i32)
        n160 = property on="ACC_IMG_DN" class="Bool"(error in=w413, "DisabledEnum"=w414) -> ()  [unwired: 1 in, 2 out]
        n161 = property on="ACC_EMAIL" class="Str"(error in=w493, "Value"=w496) -> (error out=w492:errorcluster)  [unwired: 1 in, 1 out]
        n162 = Divide(x=w510, y=w509) -> (x/y=w506:dbl)
        n163 = Divide(x=w508, y=w507) -> (x/y=w505:dbl)
        n164 = Max & Min(x=w506, y=w505) -> (min(x,y)=w504:dbl)  [unwired: 1 out]
        n165 = property on="ACC_UNIT" class="Str"(error in=w492, "Value"=w495) -> (error out=w491:errorcluster)  [unwired: 1 in, 1 out]
        n166 = property on="ACC_IMG" class="Pict"(error in=w418, "ZoomFactor"=w504, "Value"=w501) -> (error out=w503:errorcluster)  [unwired: 1 in, 1 out]
        n167 = Build Array(w451, w450, w446) -> (w449:string[][])
        n168 = property on="ACC_TITLE" class="Str"(error in=w491, "Value"=w494) -> (error out=w490:errorcluster)  [unwired: 1 in, 1 out]
        n169 = Transpose 2D Array(2D array=w449) -> (transposed array=→"ACC_ACCESS":string[][])
        n170 = Equal?(x=w433, y="NONE") -> (x = y?=w431:bool)
        n171 = property on="ACC_PSW2" class="Str"(error in=w503, "DisabledEnum"=w425) -> (error out=w512:errorcluster)  [unwired: 1 in, 1 out]
        n172 = Concatenate Strings("PERSONEL DATA VERIFICATION\nDATED  : ", w474, "\nBY     : ", w472, "\n\n================================\n\nLAST KNOWN ENTRY DATE\nPERSONEL      : ", w469, "\nSMART TAG     : ", w456, "\nACCESSIBILTY  : ", w443) -> (w471:string)
        n173 = Select(t="SUPPORTING", s=w431, f="PRODUCTION") -> (s? t:f=w429:string)
        n174 = property on="ACC_STAMP" class="Str"(error in=w490, "Value"=w433, "Caption.Text"=w429) -> (error out=w489:errorcluster)  [unwired: 1 in, 1 out]
        n175 = Get File Size(file=w488) -> (0:w487:errorcluster)  [unwired: 1 in, 2 out]
        n176 = property on="ACC_SAVE" class="Bool (strict)"(error in=w512, "DisabledEnum"=w425, "Caption.Text"="", "BoolText.Text"="SAVE RECORD" ("Boolean Text.Text")) -> (error out=w439:errorcluster)  [unwired: 1 in, 1 out]
        n177 = Unbundle By Name(w487) -> ("status"=w486:bool)
        n178 = call <vilib>:"Clear Errors.vi"("error in (no error)"=w487) -> ()  [unwired: 5 in, 2 out]
        n179 = property on="ACC_PASSPORT" class="Str"(error in=w489, "Value"=w484) -> (error out=w411:errorcluster)  [unwired: 1 in, 1 out]
        n180 = property on="ACC_TAG_ID" class="Str"("Value"=w409) -> ()  [unwired: 2 in, 2 out]
        n181 = Not(x=w486) -> (.not. x?=w423:bool)
        n182 = Empty String/Path?(string/path=w484) -> (empty?=w480:bool)
        n183 = property on="ACC_UID" class="Str"(error in=w439, "Value"=w436, "DisabledEnum"=T3."Disabled" ("Disabled"), "Text.BGColor"=u32 13816530) -> (error out=w438:errorcluster)  [unwired: 1 in, 1 out]
        n184 = property on="ACC_PASSPORT_VALID" class="Str"(error in=w411, "Value"=w412) -> (error out=w410:errorcluster)  [unwired: 1 in, 1 out]
        n185 = Select(t="NO PASSPORT", s=w480, f="NOT UPLOADED") -> (s? t:f=w478:string)
        n186 = property on="MAIN_NOTE" class="Str"(error in=w438, "Value"=w471) -> (error out=w454:errorcluster)  [unwired: 1 in, 1 out]
        n187 = Select(t="UPLOADED", s=w423, f=w478) -> (s? t:f=w482:string)
        n188 = property on="ACC_PASSPORT_STATUS" class="Bool (strict)"(error in=w410, "Value"=w423, "BoolText.Text"=w482) -> (error out=w422:errorcluster)  [unwired: 1 in, 1 out]
        n189 = property on="ACC_TAG" class="Ring (strict)"(error in=w454, "Strings []"=w459) -> (error out=w426:errorcluster)  [unwired: 1 in, 1 out]
        n190 = Select(t=T3."Enabled" ("Disabled"), s=w423, f=T3."Disabled and Grayed Out" ("Disabled")) -> (s? t:f=w419:T3)
        n191 = property on="ACC_BUTTON1" class="Bool"(error in=w426, "DisabledEnum"=w425, "Visible"=w424) -> (error out=w427:errorcluster)  [unwired: 1 in, 1 out]
        n192 = property on="ACC_PASSPORT_DN" class="Bool"(error in=w422, "DisabledEnum"=w419) -> ()  [unwired: 1 in, 2 out]
        n193 = property on="ACC_BUTTON2" class="Bool"(error in=w427, "DisabledEnum"=w425, "Visible"=w424) -> ()  [unwired: 1 in, 2 out]
      }
      frame 6 {
        w524 = T3."Disabled and Grayed Out" ("Disabled")
        # "MANAGE ACCESS PAGE SETUP"
        n194 = property on="MNG_MODULE_UPD" class="Bool"("DisabledEnum"=w524) -> (error out=w527:errorcluster)  [unwired: 2 in, 1 out]
        n195 = property on="MNG_SRC/DLT" class="Bool"(error in=w527, "DisabledEnum"=w524, "Caption.Text"="", "BoolText.Text"="SEARCH" ("Boolean Text.Text")) -> ()  [unwired: 1 in, 2 out]
      }
      frame 7, Default {
        # "FINISH SETUP"
        n196 = Unbundle(w532) -> (w554:string[], w553:string[], w534:string[], w552:string[], w551:string[], w540:path, w536:path)
        n197 = Array Subset(array=w534, index=1) -> (w533:string[])  [unwired: 1 in]
        n198 = call <vilib>:"Read JPEG File.vi"("path to JPEG file"=w540) -> ("error out"=w541:errorcluster, "image data"=w543:T8)  [unwired: 8 in, 1 out]
        n199 = property on="ACC_IMG" class="Pict"() -> (error out=w550:errorcluster, "Draw Area Size"=w542:T7)  [unwired: 2 in, 1 out]
        n200 = call <vilib>:"Draw Flattened Pixmap.vi"("image data"=w543) -> ("new picture"=w539:picture)  [unwired: 8 in]
        n201 = call <vilib>:"Clear Errors.vi"("error in (no error)"=w541) -> ()  [unwired: 5 in, 2 out]
        n202 = Get File Size(file=w536) -> (0:w537:errorcluster)  [unwired: 1 in, 2 out]
        n203 = Unbundle By Name(w537) -> ("status"=w538:bool)
        n204 = call <vilib>:"Clear Errors.vi"("error in (no error)"=w537) -> ()  [unwired: 5 in, 2 out]
        n205 = Unbundle By Name(w542) -> ("Width"=w544:u32, "Height"=w546:u32)
        n206 = Unbundle By Name(w543) -> ("Rectangle.right"=w545:i16, "Rectangle.bottom"=w547:i16)
        n207 = Not(x=w538) -> (.not. x?=w529:bool)
        n208 = Divide(x=w544, y=w545) -> (x/y=w548:dbl)
        n209 = Divide(x=w546, y=w547) -> (x/y=w549:dbl)
        n210 = Max & Min(x=w548, y=w549) -> (min(x,y)=w528:dbl)  [unwired: 1 out]
        n211 = property on="ACC_IMG" class="Pict"(error in=w550, "ZoomFactor"=w528) -> ()  [unwired: 1 in, 2 out]
        n212 = Bundle(w554, w553, w533, w552, w551, "new picture"=w539, w528, w529) -> (w531:T9)  [unwired: 1 in]
      }
    }
  }
  n213 = while {
    shift-right: [w560] -> _
    shift-left: w1 -> [w559]
    tunnel: w2 -> [w558]
    shift-right: [w556] -> _
    shift-left: w1 -> [w557]
    stop <- w563 stop-if-true
    # "MAIN LOOP"
    n214 = event shown="[9] \"ACC_SAVE\": Value Change" {
      selector: _ -> [_ _ _ _ _ _ _ _ _ _]
      dyn-events: _ -> [_ _ _ _ _ _ _ _ _ _]
      timeout: 10 -> [_ _ _ _ _ _ _ _ _ _]
      tunnel: [_ w634 _ _ _ _ _ _ _ _] -> w563
      tunnel: [_ _ _ w646 _ _ _ _ _ _] -> w562
      tunnel: [w631 w633 w639 w645 w724 w735 w745 w758 _ _] -> w561
      tunnel: w559 -> [w631 w633 w639 w644 w724 w735 w745 w758 _ _]
      tunnel: w558 -> [_ _ _ w643 _ _ _ _ _ w775]
      tunnel: w557 -> [w630 w632 w638 w642 w723 w734 w744 w756 _ _]
      tunnel: [w630 w632 w638 w641 w723 w734 w744 w756 _ _] -> w556
      event Timeout {
        n215 = event-data() -> ()  [unwired: 1 in, 3 out]
      }
      event "MAIN_CLOSE": Value Change {
        n216 = event-data() -> ("OldVal"=w635:bool, "NewVal"=w637:bool)  [unwired: 1 in, 4 out]
        n217 = Not(x=w637) -> (.not. x?=w636:bool)
        n218 = And(x=w635, y=w636) -> (x .and. y?=w634:bool)
      }
      event "MAIN_TAB": Value Change {
        n219 = event-data() -> ()  [unwired: 1 in, 6 out]
      }
      event "ACC_OPTION": Value Change {
        n220 = event-data() -> ("NewVal"=w647:enum32{"Item 0", "Item 1", "Item 2"})  [unwired: 1 in, 5 out]
        n221 = case shown="\"Item 0\", Default" w647 {
          tunnel: [TRUE TRUE TRUE] -> w646
          tunnel: [w649 T9 {[], [], [], [], [], "new picture"=bytes[0], 0.0, FALSE} w700] -> w645
          tunnel: w644 -> [_ _ w700]
          tunnel: w643 -> [w651 w680 w699]
          tunnel: w642 -> [w649 w681 w697]
          tunnel: [w649 w681 w697] -> w641
          tunnel: [T3."Enabled" ("Disabled") w667 T3."Disabled and Grayed Out" ("Disabled")] -> w640
          frame "Item 0", Default {
            w654 = ""
            w656 = T3."Disabled and Grayed Out" ("Disabled")
            # "MY ACCOUNT"
            n222 = Unbundle(w651) -> (w650:string[])  [unwired: 1 out]
            n223 = Index Array(array=w650) -> (element=w662:string)  [unwired: 1 in]
            n224 = property on="ACC_UID" class="Str"("Value"=w662, "Text.BGColor"=u32 13816530, "DisabledEnum"=T3."Disabled" ("Disabled")) -> (error out=w666:errorcluster)  [unwired: 2 in, 1 out]
            n225 = property on="ACC_PSW1" class="Str"(error in=w666, "Visible"=TRUE, "DisabledEnum"=T3."Enabled" ("Disabled"), "Value"=w654) -> (error out=w665:errorcluster)  [unwired: 1 in, 1 out]
            n226 = property on="ACC_PSW2" class="Str"(error in=w665, "Visible"=TRUE, "DisabledEnum"=w656, "Value"=w654) -> (error out=w658:errorcluster)  [unwired: 1 in, 1 out]
            n227 = property on="ACC_BUTTON1" class="Bool"(error in=w658, "BoolText.Text"="CHANGE PASSWORD", "DisabledEnum"=w656) -> (error out=w657:errorcluster)  [unwired: 1 in, 1 out]
            n228 = property on="ACC_BUTTON2" class="Bool"(error in=w657, "DisabledEnum"=w656, "Visible"=TRUE) -> ()  [unwired: 1 in, 2 out]
          }
          frame "Item 1" {
            w670 = T3."Enabled" ("Disabled")
            w669 = T3."Disabled and Grayed Out" ("Disabled")
            # "SEARCH ACCOUNT"
            n229 = Unbundle(w680) -> (w679:string[])  [unwired: 1 out]
            n230 = Index Array(array=w679, index=3) -> (element=w673:string)
            n231 = Match Pattern(string=w673, regular expression="W") -> (offset past match=w671:i32)  [unwired: 1 in, 3 out]
            n232 = Match Pattern(string=w673, regular expression="D") -> (offset past match=w676:i32)  [unwired: 1 in, 3 out]
            n233 = property on="ACC_PSW1" class="Str"("Value"="", "DisabledEnum"=w669) -> (error out=w691:errorcluster)  [unwired: 2 in, 1 out]
            n234 = Greater Or Equal To 0?(x=w671) -> (x >= 0?=w668:bool)
            n235 = Greater Or Equal To 0?(x=w676) -> (x >= 0?=w675:bool)
            n236 = property on="ACC_PSW2" class="Str"(error in=w691, "Value"="", "Visible"=FALSE, "DisabledEnum"=w669) -> (error out=w690:errorcluster)  [unwired: 1 in, 1 out]
            n237 = property on="ACC_BUTTON1" class="Bool"(error in=w690, "BoolText.Text"="SEARCH") -> (error out=w689:errorcluster)  [unwired: 1 in, 1 out]
            n238 = property on="ACC_BUTTON2" class="Bool"(error in=w689, "Visible"=w675) -> (error out=w686:errorcluster)  [unwired: 1 in, 1 out]
            n239 = property on="ACC_UID" class="Str"(error in=w686, "Value"="", "DisabledEnum"=w670, "Text.BGColor"=u32 16777226) -> (error out=w674:errorcluster)  [unwired: 1 in, 1 out]
            n240 = Select(t=w670, s=w668, f=w669) -> (s? t:f=w667:T3)
            n241 = case shown="True" w675 {
              tunnel: w674 -> [_ w695]
              frame False {
                # "DO NOTHING"
              }
              frame True {
                # "CHANGE BOOL.TEXT"
                n242 = property on="ACC_BUTTON2" class="Bool"(error in=w695, "BoolText.Text"="DELETE") -> ()  [unwired: 1 in, 2 out]
              }
            }
          }
          frame "Item 2" {
            w702 = ""
            # "CREATE ACCOUNT"
            n243 = Unbundle(w699) -> (w698:string[])  [unwired: 1 out]
            n244 = Index Array(array=w698, index=3) -> (element=w715:string)
            n245 = Match Pattern(string=w715, regular expression="W") -> (offset past match=w713:i32)  [unwired: 1 in, 3 out]
            n246 = Greater Or Equal To 0?(x=w713) -> (x >= 0?=w712:bool)
            n247 = case shown="False" w712 {
              tunnel: [T3."Disabled and Grayed Out" ("Disabled") T3."Enabled" ("Disabled")] -> w709
              tunnel: [FALSE TRUE] -> w710
              tunnel: [u32 15000804 u32 16777226] -> w708
              frame False {
                # "NOT ACCESSIBLE"
              }
              frame True {
                # "ACCESSIBLE"
              }
            }
            n248 = property on="ACC_UID" class="Str"("Value"=w702, "DisabledEnum"=w709, "Text.BGColor"=w708) -> (error out=w711:errorcluster)  [unwired: 2 in, 1 out]
            n249 = property on="ACC_PSW1" class="Str"(error in=w711, "Value"=w702, "DisabledEnum"=w709) -> (error out=w707:errorcluster)  [unwired: 1 in, 1 out]
            n250 = property on="ACC_PSW2" class="Str"(error in=w707, "Visible"=w710, "Value"=w702) -> (error out=w706:errorcluster)  [unwired: 1 in, 1 out]
            n251 = property on="ACC_BUTTON2" class="Bool"(error in=w706, "Visible"=FALSE) -> (error out=w704:errorcluster)  [unwired: 1 in, 1 out]
            n252 = property on="ACC_BUTTON1" class="Bool"(error in=w704, "BoolText.Text"="CREATE ACCOUNT") -> ()  [unwired: 1 in, 2 out]
          }
        }
        n253 = property on="ACC_PASSPORT_UP" class="Bool"("DisabledEnum"=w640) -> ()  [unwired: 2 in, 2 out]
        n254 = property on="ACC_IMG_UP" class="Bool"("DisabledEnum"=w640) -> ()  [unwired: 2 in, 2 out]
        n255 = property on="ACC_NAME" class="Str"("DisabledEnum"=w640) -> ()  [unwired: 2 in, 2 out]
        n256 = property on="ACC_EMAIL" class="Str"("DisabledEnum"=w640) -> ()  [unwired: 2 in, 2 out]
        n257 = property on="ACC_UNIT" class="Str"("DisabledEnum"=w640) -> ()  [unwired: 2 in, 2 out]
        n258 = property on="ACC_TITLE" class="Str"("DisabledEnum"=w640) -> ()  [unwired: 2 in, 2 out]
        n259 = property on="ACC_STAMP" class="Str"("DisabledEnum"=w640) -> ()  [unwired: 2 in, 2 out]
        n260 = property on="ACC_PASSPORT" class="Str"("DisabledEnum"=w640) -> ()  [unwired: 2 in, 2 out]
        n261 = property on="ACC_PASSPORT_VALID" class="Str"("DisabledEnum"=w640) -> ()  [unwired: 2 in, 2 out]
      }
      event "ACC_PSW1": Value Change {
        n262 = event-data() -> ("NewVal"=w731:string)  [unwired: 1 in, 5 out]
        n263 = property on="Item 1" class="Bool (strict)"() -> ("Value"=w726:bool)  [unwired: 2 in, 2 out]
        n264 = Empty String/Path?(string/path=w731) -> (empty?=w730:bool)
        n265 = Not(x=w726) -> (.not. x?=w725:bool)
        n266 = Not(x=w730) -> (.not. x?=w729:bool)
        n267 = And(x=w725, y=w729) -> (x .and. y?=w728:bool)
        n268 = Select(t=T3."Enabled" ("Disabled"), s=w728, f=T3."Disabled and Grayed Out" ("Disabled")) -> (s? t:f=w727:T3)
        n269 = property on="ACC_PSW2" class="Str"("DisabledEnum"=w727) -> ()  [unwired: 2 in, 2 out]
      }
      event "ACC_UID": Value Change {
        n270 = event-data() -> ("NewVal"=w743:string)  [unwired: 1 in, 5 out]
        n271 = Empty String/Path?(string/path=w743) -> (empty?=w742:bool)
        n272 = property on="Item 1" class="Bool (strict)"() -> ("Value"=w740:bool)  [unwired: 2 in, 2 out]
        n273 = Not(x=w742) -> (.not. x?=w741:bool)
        n274 = And(x=w741, y=w740) -> (x .and. y?=w739:bool)
        n275 = Select(t=T3."Enabled" ("Disabled"), s=w739, f=T3."Disabled and Grayed Out" ("Disabled")) -> (s? t:f=w736:T3)
        n276 = property on="ACC_BUTTON1" class="Bool"("DisabledEnum"=w736) -> ()  [unwired: 2 in, 2 out]
      }
      event "ACC_PSW2": Value Change {
        n277 = event-data() -> ("NewVal"=w755:string)  [unwired: 1 in, 5 out]
        n278 = Empty String/Path?(string/path=w755) -> (empty?=w754:bool)
        n279 = property on="Item 1" class="Bool (strict)"() -> ("Value"=w753:bool)  [unwired: 2 in, 2 out]
        n280 = Not(x=w753) -> (.not. x?=w752:bool)
        n281 = Not(x=w754) -> (.not. x?=w751:bool)
        n282 = And(x=w752, y=w751) -> (x .and. y?=w750:bool)
        n283 = Select(t=T3."Enabled" ("Disabled"), s=w750, f=T3."Disabled and Grayed Out" ("Disabled")) -> (s? t:f=w746:T3)
        n284 = property on="ACC_BUTTON1" class="Bool"("DisabledEnum"=w746) -> (error out=w747:errorcluster)  [unwired: 2 in, 1 out]
        n285 = property on="ACC_BUTTON2" class="Bool"(error in=w747, "DisabledEnum"=w746) -> ()  [unwired: 1 in, 2 out]
      }
      event "ACC_TAG": Value Change {
        n286 = event-data() -> ()  [unwired: 1 in, 6 out]
        n287 = Unbundle(w758) -> (w760:string[])  [unwired: 7 out]
        n288 = Index Array(array=w760, index="ACC_TAG") -> (element=w759:string)
        n289 = property on="ACC_TAG_ID" class="Str"("Value"=w759) -> ()  [unwired: 2 in, 2 out]
      }
      event "ACC_NAME": Value Change {
        n290 = event-data() -> ("NewVal"=w768:string)  [unwired: 1 in, 5 out]
        n291 = Empty String/Path?(string/path=w768) -> (empty?=w767:bool)
        n292 = Not(x=w767) -> (.not. x?=w763:bool)
        n293 = property on="Item 1" class="Bool (strict)"() -> ("Value"=w764:bool)  [unwired: 2 in, 2 out]
        n294 = And(x=w764, y=w763) -> (x .and. y?=w762:bool)
        n295 = Select(t=T3."Enabled" ("Disabled"), s=w762, f=T3."Disabled and Grayed Out" ("Disabled")) -> (s? t:f=w761:T3)
        n296 = property on="ACC_BUTTON2" class="Bool"("DisabledEnum"=w761) -> ()  [unwired: 2 in, 2 out]
      }
      event "ACC_SAVE": Value Change {
        n297 = event-data() -> ("OldVal"=w771:bool, "NewVal"=w776:bool)  [unwired: 1 in, 4 out]
        n298 = property on="ACC_NAME" class="Str"() -> ("Value"=w774:string)  [unwired: 2 in, 2 out]
        n299 = Empty String/Path?(string/path=w774) -> (empty?=w773:bool)
        n300 = Not(x=w776) -> (.not. x?=w772:bool)
        n301 = Not(x=w773) -> (.not. x?=w770:bool)
        n302 = Compound Arithmetic op=AND(w770, w771, w772) -> (w769:bool)
        n303 = case shown="True" w769 {
          tunnel: w775 -> [_ w779]
          frame False {
            # "DO NOTHING"
          }
          frame True {
            # "EXEC QUERY"
            n304 = Unbundle(w779) -> (w778:path[])  [unwired: 1 out]
            n305 = Index Array(array=w778) -> (element=w777:path)  [unwired: 1 in]
            n306 = call-poly <vilib>:"DB Tools Open Connection.vi"("connection information"=w777) -> ()  [unwired: 7 in, 2 out]
          }
        }
      }
    }
    n307 = case shown="True" w562 {
      tunnel: w561 -> [w565 w586]
      tunnel: [w565 w586] -> w560
      frame False {
        # "DO NOTHING"
      }
      frame True {
        w568 = T3."Disabled and Grayed Out" ("Disabled")
        w569 = T3."Enabled" ("Disabled")
        # "DISPLAY FIELDS - ACCOUNT TAB"
        n308 = Unbundle(w586) -> (w617:string[], w605:string[], w595:string[], w594:string[], "new picture"=w574:picture, w585:dbl, w570:bool)  [unwired: 1 out]
        n309 = Array Subset(array=w605, index=1) -> (w604:string[])  [unwired: 1 in]
        n310 = Array Subset(array=w595, index=1) -> (w596:string[])  [unwired: 1 in]
        n311 = Array Subset(array=w594, index=1) -> (w598:string[])  [unwired: 1 in]
        n312 = Index Array(array=w617, index #1=1 ("index")) -> (element #1=w615:string, element #2=w610:string, element #3=w609:string, element #4=w608:string, element #5=w584:string, element #6=w587:string, element #7=w590:string)  [unwired: 6 in]
        n313 = property on="ACC_NAME" class="Str"("Value"=w615) -> (error out=w614:errorcluster)  [unwired: 2 in, 1 out]
        n314 = Array Size(array=w596) -> (size(s)=w603:i32)
        n315 = for {
          N: w603 -> [_]
          tunnel: w596 -> [w629]
          tunnel: [w624] -> w601 mode=indexing
          tunnel: [w621] -> w602 mode=indexing
          i -> [w623]
          # "REPLACING '_' WITH %s"
          n316 = Increment(x=w623) -> (x+1=w622:i32)
          n317 = Index Array(array=w629, index=w623) -> (element=w628:string)
          n318 = call <vilib>:"Space Constant.vi"() -> ("String"=w626:string)
          n319 = Search and Replace String(replace all?=TRUE, input string=w628, search string="_", replace string=w626) -> (result string=w624:string)  [unwired: 4 in, 3 out]
          n320 = Number To Decimal String(number=w622) -> (decimal integer string=w621:string)  [unwired: 1 in]
        }
        n321 = case shown="\"\"" w584 {
          tunnel: ["NO DATA" ("y") "SUPPORTING" "PRODUCTION"] -> w583
          frame "" {
          }
          frame "NONE" {
          }
          frame Default {
          }
        }
        n322 = property on="ACC_EMAIL" class="Str"(error in=w614, "Value"=w610) -> (error out=w613:errorcluster)  [unwired: 1 in, 1 out]
        n323 = property on="ACC_UNIT" class="Str"(error in=w613, "Value"=w609) -> (error out=w612:errorcluster)  [unwired: 1 in, 1 out]
        n324 = property on="ACC_TITLE" class="Str"(error in=w612, "Value"=w608) -> (error out=w611:errorcluster)  [unwired: 1 in, 1 out]
        n325 = Build Array(w602, w601, w598) -> (w600:string[][])
        n326 = property on="ACC_STAMP" class="Str"(error in=w611, "Value"=w584, "Caption.Text"=w583) -> (error out=w607:errorcluster)  [unwired: 1 in, 1 out]
        n327 = Transpose 2D Array(2D array=w600) -> (transposed array=w593:string[][])
        n328 = property on="ACC_IMG" class="Pict"("Value"=w574, "ZoomFactor"=w585) -> ()  [unwired: 2 in, 2 out]
        n329 = Empty String/Path?(string/path=w587) -> (empty?=w579:bool)
        n330 = property on="ACC_PASSPORT" class="Str"(error in=w607, "Value"=w587) -> (error out=w591:errorcluster)  [unwired: 1 in, 1 out]
        n331 = And(x=w570, y=w579) -> (x .and. y?=w582:bool)
        n332 = property on="ACC_PASSPORT_VALID" class="Str"(error in=w591, "Value"=w590) -> (error out=w589:errorcluster)  [unwired: 1 in, 1 out]
        n333 = Select(t="NO PASSPORT" ("f"), s=w579, f="NOT UPLOADED") -> (s? t:f=w576:string)
        n334 = Select(t="UPLOADED", s=w582, f=w576) -> (s? t:f=w580:string)
        n335 = Equal?(x=picture data[5B] ("new picture"), y=w574) -> (x = y?=w572:bool)
        n336 = property on="ACC_PASSPORT_STATUS" class="Bool (strict)"(error in=w589, "Value"=w570, "BoolText.Text"=w580) -> (error out=w588:errorcluster)  [unwired: 1 in, 1 out]
        n337 = property on="ACC_TAG" class="Ring (strict)"(error in=w588, "Strings []"=w604) -> (error out=w592:errorcluster)  [unwired: 1 in, 1 out]
        n338 = property on="ACC_ACCESS" class="Tbl (strict)"(error in=w592, "Value"=w593) -> (error out=w575:errorcluster)  [unwired: 1 in, 1 out]
        n339 = Select(t=w568, s=w572, f=w569) -> (s? t:f=w571:T3)
        n340 = property on="ACC_IMG_DN" class="Bool"(error in=w575, "DisabledEnum"=w571) -> (error out=w566:errorcluster)  [unwired: 1 in, 1 out]
        n341 = Select(t=w569, s=w570, f=w568) -> (s? t:f=w567:T3)
        n342 = property on="ACC_PASSPORT_DN" class="Bool"(error in=w566, "DisabledEnum"=w567) -> ()  [unwired: 1 in, 2 out]
      }
    }
  }
